vi "API Build Command.vi"(0 "Action":string, 5 "Double":dbl[](array[numeric]), 7 "Integer":i32[](array[numeric]), 9 "Boolean":bool[](array[boolean]), 11 "String":string[](array[string])) -> (8 "PIM.API.Command.Unique":T1)   [LabVIEW 2011]
uses:
  Controls/PIM.API.Command.Unique.ctl
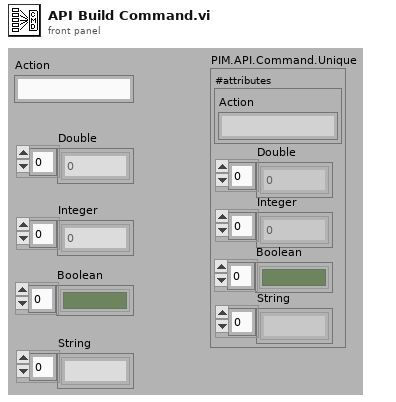
[diagram p1: front panel]
types:
  T1 = typedef "PIM.API.Command.Unique.ctl" = cluster{"#attributes":cluster{"Action":string}, "Double":dbl[], "Integer":i32[], "Boolean":bool[], "String":string[]}
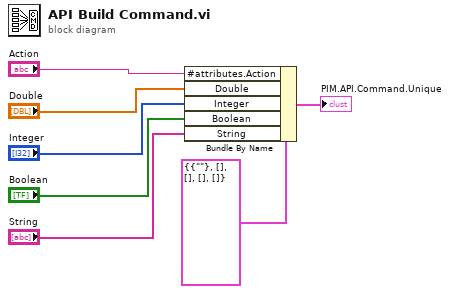
[diagram p0: block diagram]
diagram:
  n1 = Bundle By Name(cluster=T1 {"#attributes"={"Action"=""}, "Double"=[], "Integer"=[], "Boolean"=[], "String"=[]} ("PIM.API.Command.Unique"), "#attributes.Action"="Action", "Double"="Double", "Integer"="Integer", "Boolean"="Boolean", "String"="String") -> (→"PIM.API.Command.Unique":T1)
